vi "Create Subscription.vi"(8 "error in (no error)":errorcluster, 9 "Protocol":T1, 10 "Endpoint":string, 11 "Topic":refnum<class "Topic.lvclass">) -> (0 "error out":errorcluster, 3 "Subscription out":refnum<class "Subscription.lvclass">)   [LabVIEW 2015, in "NI_AWS_SNS.lvlib" / "Subscription.lvclass"]
uses:
  Subscription.lvclass
  Subscription Protocol.ctl
  Topic/Topic.lvclass
  Core/HTTP Request/Request Options.ctl
  Core/HTTP Request/Name Value Pair.ctl
  Core/ARN/ARN.lvclass/ARN.ctl
  Core/HTTP Request/HTTP Request.lvclass/HTTP Request.ctl
  Subscription.lvclass/Subscription.ctl
  Core/ARN/Read ARN.vi
  Core/HTTP Request/Read Credentials.vi
  Core/HTTP Request/Read Region.vi
  Write Topic.vi
  Write Protocol.vi
  Write Endpoint.vi
  Write Owner.vi
  Core/HTTP Request/HTTP Request.lvclass
  Core/ARN/ARN.lvclass
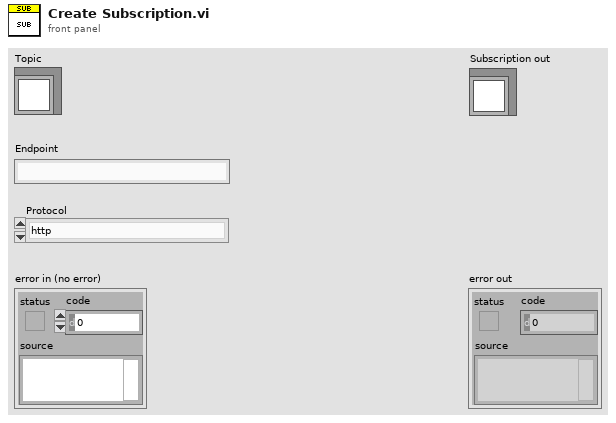
[diagram p1: front panel]
types:
  T1 = typedef "NI_AWS_SNS.lvlib/Subscription.lvclass/Subscription Protocol.ctl" = enum16{"http", "https", "email", "email-json", "sms", "sqs", "application", "lambda"}
  T2 = typedef "NI_AWS_Core.lvlib/HTTP Request.lvclass/Name Value Pair.ctl" = cluster{"name":string, "value":string}
  T3 = typedef "NI_AWS_Core.lvlib/HTTP Request.lvclass/Request Options.ctl" = cluster{"request headers":T2[], "request parameters":T2[], "request body":string, "ignore region":bool}
  T4 = typedef "NI_AWS_Core.lvlib/HTTP Request.lvclass/AWS Credentials.ctl" = cluster{"Access Key":string, "Secret Key":string}
  T5 = typedef "NI_AWS_Core.lvlib/HTTP Request.lvclass/Region.ctl" = enum16{"us-east-1", "us-east-2", "us-west-1", "us-west-2", "ap-northeast-1", "ap-northeast-2", "ap-southeast-1", "ap-southeast-2", "ca-central-1", "eu-central-1", "eu-west-1", "eu-west-2", "sa-east-1"}
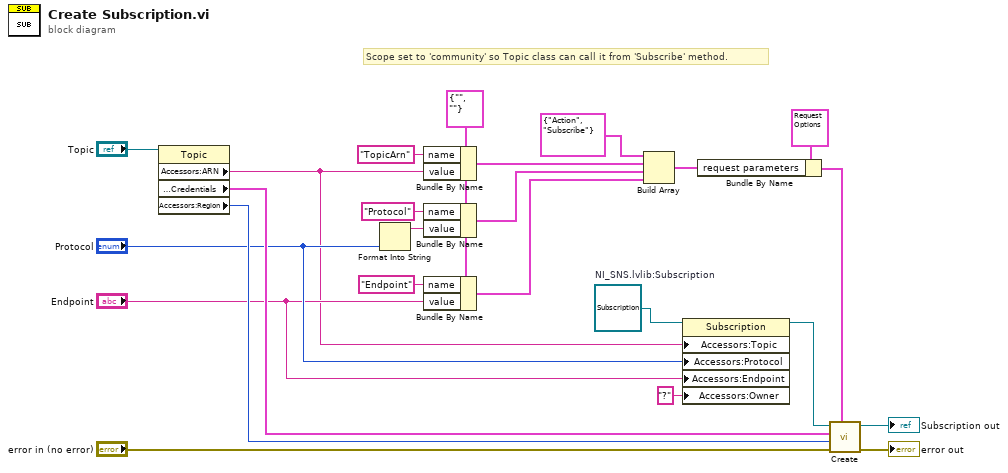
[diagram p0: block diagram]
diagram:
  w6 = refnum<class "Subscription.lvclass"> refnum  # NI_SNS.lvlib:Subscription
  w16 = T2 {"name"="", "value"=""} ("element")
  # "Scope set to 'community' so Topic class can call it from 'Subscribe' method."
  n1 = property class="Topic"(reference="Topic") -> ("Accessors:ARN"=w1:string, "Accessors:Credentials"=w7:T4, "Accessors:Region"=w8:T5)  [unwired: 1 in, 2 out]
  n2 = Format Into String("Protocol") -> (resulting string=w13:string)  [unwired: 3 in, 1 out]
  n3 = Bundle By Name(cluster=w16, "name"="TopicArn", "value"=w1) -> (w22:T2)
  n4 = Bundle By Name(cluster=w16, "name"="Protocol", "value"=w13) -> (w15:T2)
  n5 = Bundle By Name(cluster=w16, "name"="Endpoint", "value"="Endpoint") -> (w14:T2)
  n6 = Build Array(T2 {"name"="Action", "value"="Subscribe"} ("Name Value Pair"), w22, w15, w14) -> (w21:T2[])
  n7 = property class="Subscription"(reference=w6, "Accessors:Topic"=w1, "Accessors:Protocol"="Protocol", "Accessors:Endpoint"="Endpoint", "Accessors:Owner"="?" ("Owner")) -> (reference out=w5:refnum<class "Subscription.lvclass">)  [unwired: 1 in, 1 out]
  n8 = Bundle By Name(cluster=T3 {"request headers"=[], "request parameters"=[{"name"="Action", "value"="ListQueues"}], "request body"="", "ignore region"=FALSE} ("Request Options"), "request parameters"=w21) -> (w10:T3)
  n9 = call "Create.vi"("Request Options"=w10, "error in (no error)"="error in (no error)", "Region"=w8, "AWS Credentials"=w7, "ARN in"=w5) -> ("error out"=→"error out":errorcluster, "ARN out"=→"Subscription out":refnum<class "Subscription.lvclass">)  [unwired: 5 in]
